vi "Calculate New Status.vi"(8 "error in (no error)":errorcluster, 10 "New Status":T1, 11 "abs_Parallel in":refnum<class "bt_Parallel.lvclass">) -> (0 "error out":errorcluster, 2 "Overall Status":T1, 3 "abs_Parallel out":refnum<class "bt_Parallel.lvclass">)   [LabVIEW 2021, in "BT.lvlib" / "bt_Parallel.lvclass"]
uses:
  bt_Parallel.lvclass
  C:/Users/Tim/Documents/GitHub/LV_Behaviour_Tree/Source/Support/Nodes/Composites/abs_Composite/bt_Composite.lvclass
  abs_Node/Status.ctl
  abs_Composite/bt_Composite.lvclass/bt_Composite.ctl
  bt_Parallel.lvclass/bt_Parallel.ctl
  abs_Composite/Properties/Read Index.vi
  Properties/Read Status Calculation.vi
  abs_Node/bt_Node.lvclass
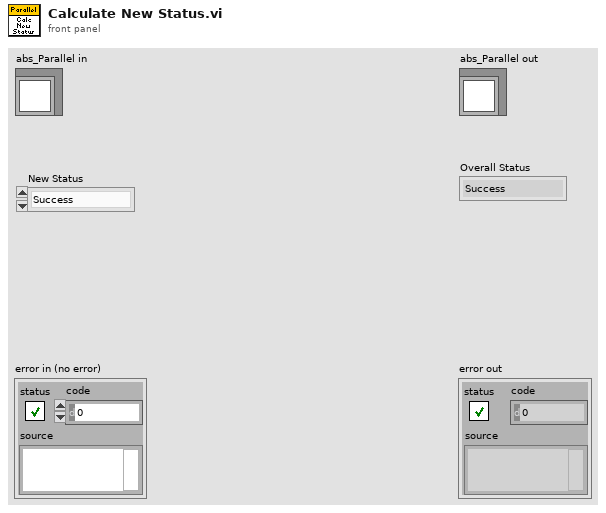
[diagram p1: front panel]
types:
  T1 = typedef "BT.lvlib/bt_Node.lvclass/Status.ctl" = enum16{"Success", "Failure", "Running"}
  T2 = typedef "BT.lvlib/bt_Parallel.lvclass/Status Calculation.ctl" = enum16{"Succeed on All Succeed", "Failure on All Failure", "Succeed on Any Succeed", "Failure on Any Failure"}
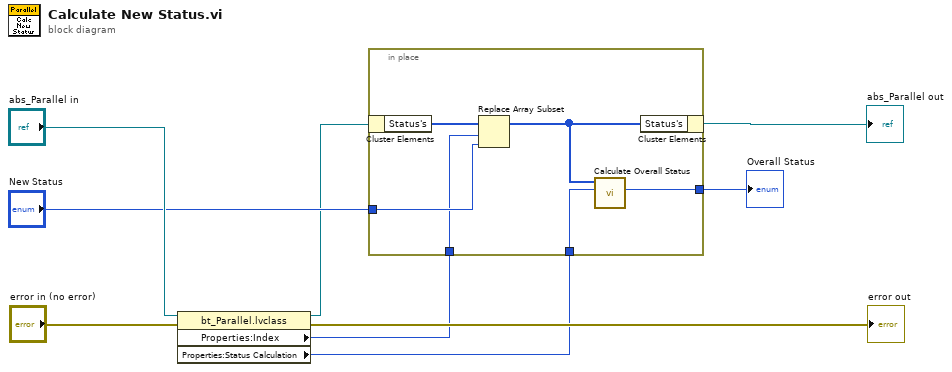
[diagram p0: block diagram]
diagram:
  n1 = property class="bt_Parallel.lvclass"(reference="abs_Parallel in", error in="error in (no error)") -> (reference out=w4:refnum<class "bt_Parallel.lvclass">, error out=→"error out":errorcluster, "Properties:Index"=w5:i32, "Properties:Status Calculation"=w2:T2)
  n2 = in-place {
    in-place-border: "New Status" -> [w15]
    in-place-border: w5 -> [w14]
    in-place-border: w2 -> [w11]
    in-place-border: [w10] -> w1
    n3 = in-place-cluster #1(w4) -> ("Status's"=w13:T1[])
    n4 = Replace Array Subset(array=w13, new element=w15, index=w14) -> (w12:T1[])
    n5 = call "Calculate Overall Status.vi"("Status Calculation"=w11, "Status's"=w12) -> ("Overall Status"=w10:T1)  [unwired: 9 in]
    n6 = in-place-cluster #1("Status's"=w12) -> (→"abs_Parallel out":refnum<class "bt_Parallel.lvclass">)
  }
  "Overall Status" <- w1
